vi "习7.1.vi"() -> ()   [LabVIEW 2017]
uses:
  <vilib>/measure/NI_MABase.lvlib
panel:
  in  "phase":dbl caption="相位" format="%.2p"
  out "XY图":cluster{"Y":dbl[], "Y":dbl[]}(graph)
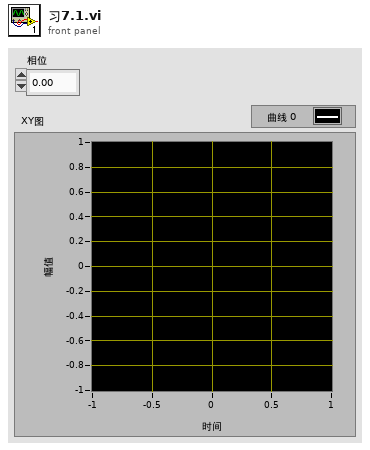
[diagram p1: front panel]
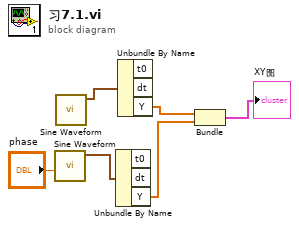
[diagram p0: block diagram]
diagram:
  n1 = call <vilib>:"Sine Waveform.vi"("phase"="phase") -> ("signal out"=w6:waveform(dbl))  [unwired: 9 in, 1 out]
  n2 = call <vilib>:"Sine Waveform.vi"() -> ("signal out"=w5:waveform(dbl))  [unwired: 10 in, 1 out]
  n3 = Unbundle By Name(w6) -> ("Y"=w4:dbl[])  [unwired: 2 out]
  n4 = Unbundle By Name(w5) -> ("Y"=w3:dbl[])  [unwired: 2 out]
  n5 = Bundle("Y"=w3, "Y"=w4) -> (→"XY图":cluster{"Y":dbl[], "Y":dbl[]})  [unwired: 1 in]
